vi "remove_negative.vi"(1 "input array":dbl[](array[numeric])) -> (0 "output array":dbl[](array[numeric]))   [LabVIEW 2012]
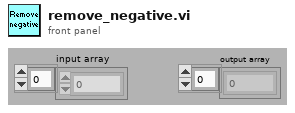
[diagram p1: front panel]
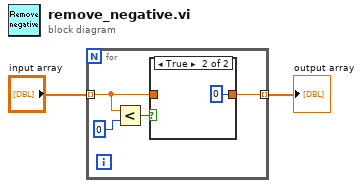
[diagram p0: block diagram]
diagram:
  n1 = for {
    tunnel: "input array" -> [w3] mode=indexing
    tunnel: [w4] -> w2 mode=indexing
    n2 = Less?(x=w3, y=0) -> (x < y?=w6:bool)
    n3 = case shown="True" w6 {
      tunnel: [w7 0] -> w4
      tunnel: w3 -> [w7 _]
      frame False {
      }
      frame True {
      }
    }
  }
  "output array" <- w2
